vi "Buttons2.vi"() -> ()   [LabVIEW 2019]
panel:
  in  "LPB":bool
  in  "SPB":bool
  in  "LPA":bool
  in  "SPA":bool
  in  "Simulation":bool=TRUE
  in  "Array":bool[](array[boolean])=[FALSE, FALSE, FALSE, FALSE, FALSE, FALSE, FALSE, FALSE]
  in  "B":bool
  in  "A":bool
  in  "Exit":bool
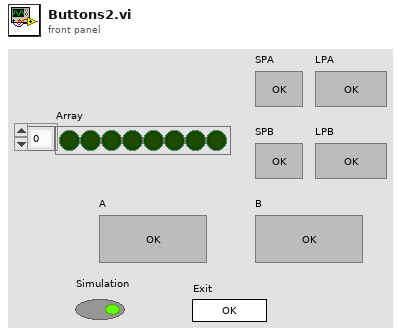
[diagram p1: front panel]
types:
  T1 = enum32{"Invalid", "Standard", "Closed", "Hidden", "Minimized", "Maximized"}
  T2 = enum32{"invalid app kind", "Development System", "Run Time System", "Student Edition", "Embedded LabVIEW", "Evaluation", "Custom"}
  T3 = cluster{"Core":cluster{"Current VI Reference":refnum<vi>, "Close Panel on Exit?":bool}, "A":bool, "B":bool, "Array":bool[], "NA":i32, "NB":i32}
  T4 = cluster{"Current VI Reference":refnum<vi>, "Close Panel on Exit?":bool}
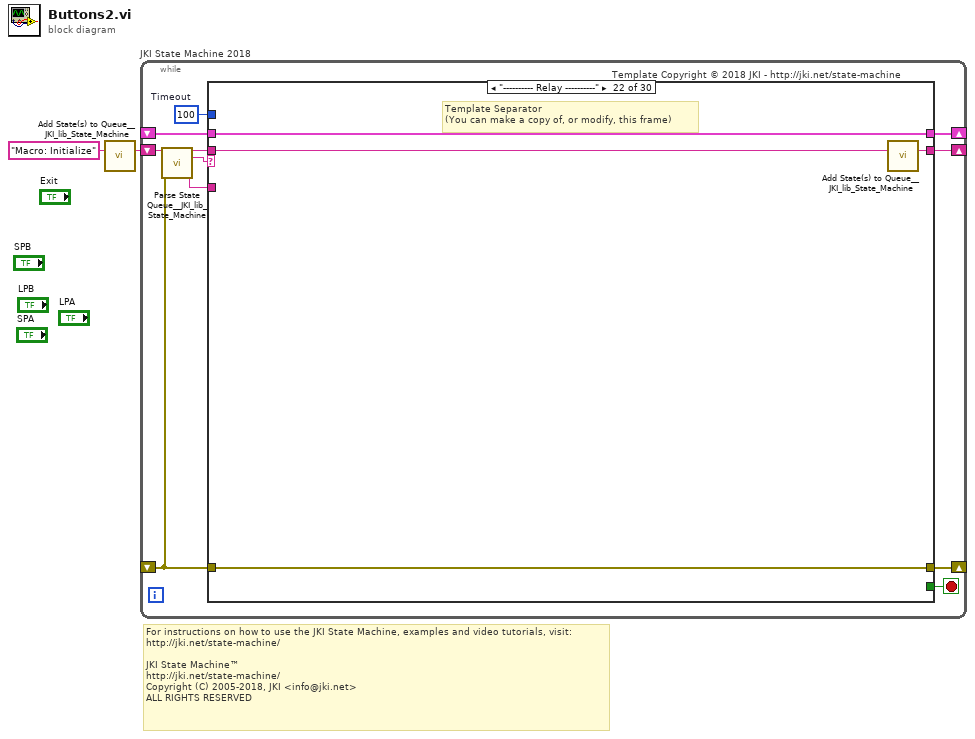
[diagram p0: block diagram]
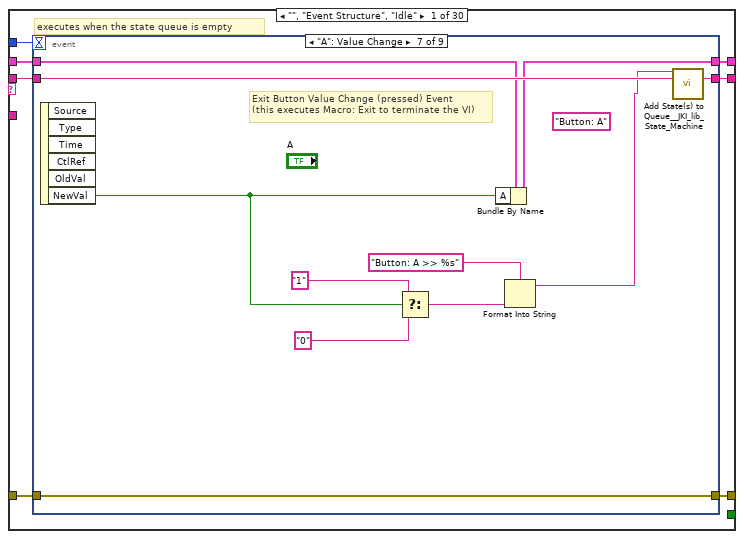
[diagram p2: hidden frame]
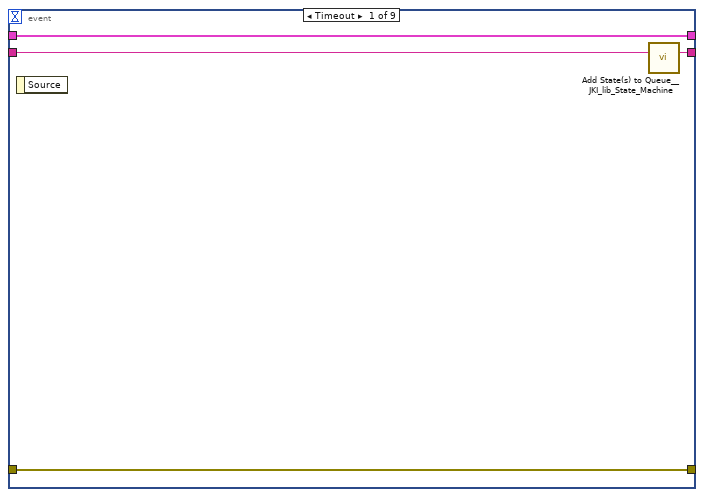
[diagram p3: hidden frame]
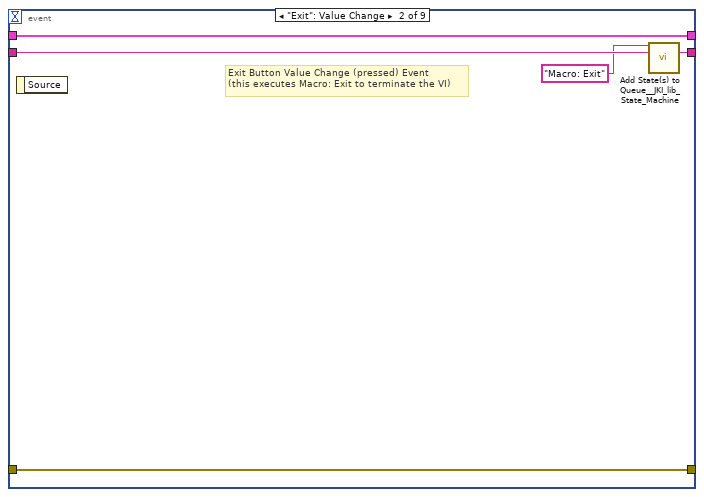
[diagram p4: hidden frame]
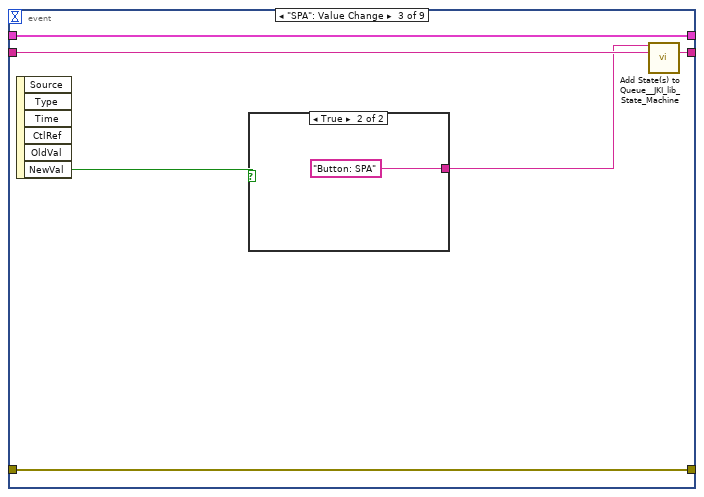
[diagram p5: hidden frame]
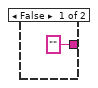
[diagram p6: hidden frame]
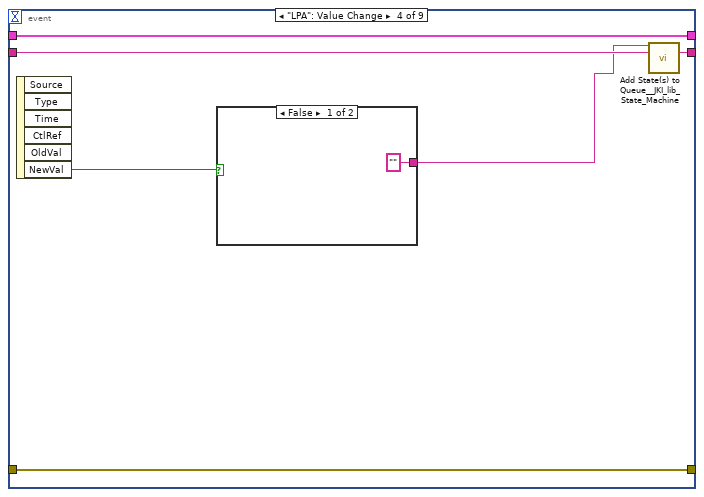
[diagram p7: hidden frame]
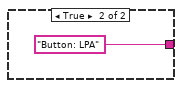
[diagram p8: hidden frame]
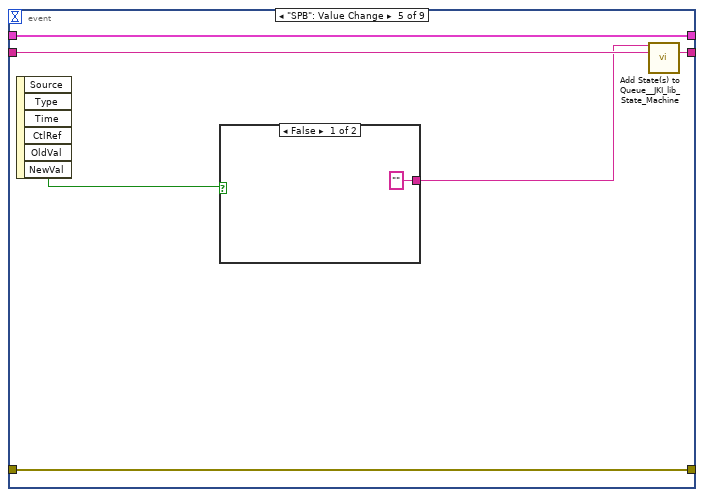
[diagram p9: hidden frame]
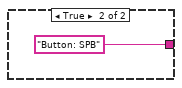
[diagram p10: hidden frame]
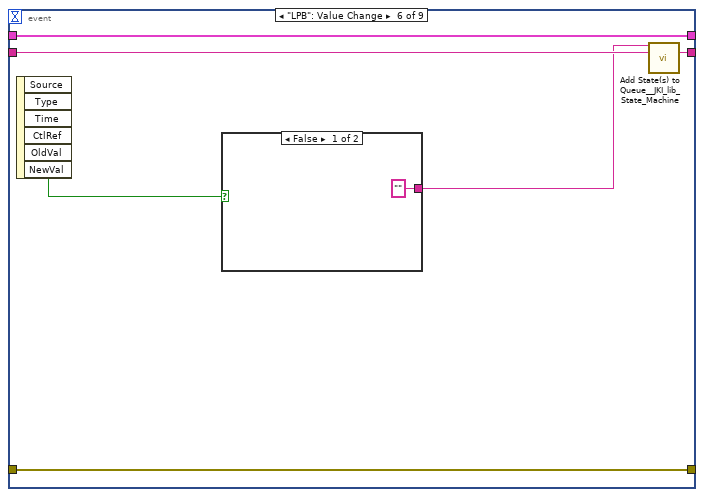
[diagram p11: hidden frame]
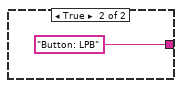
[diagram p12: hidden frame]
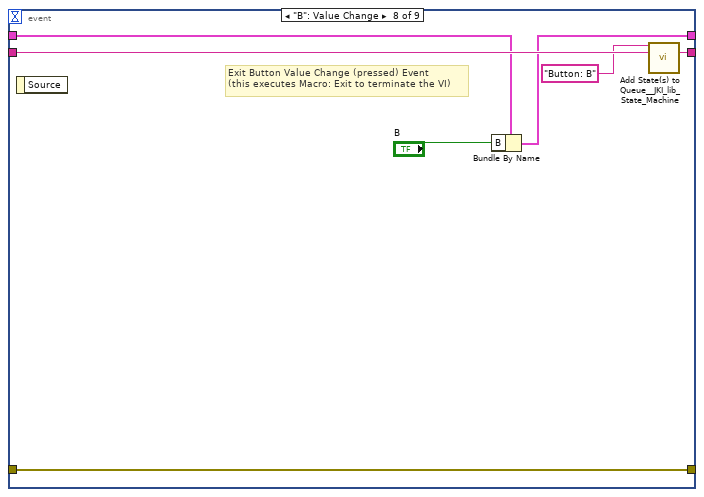
[diagram p13: hidden frame]
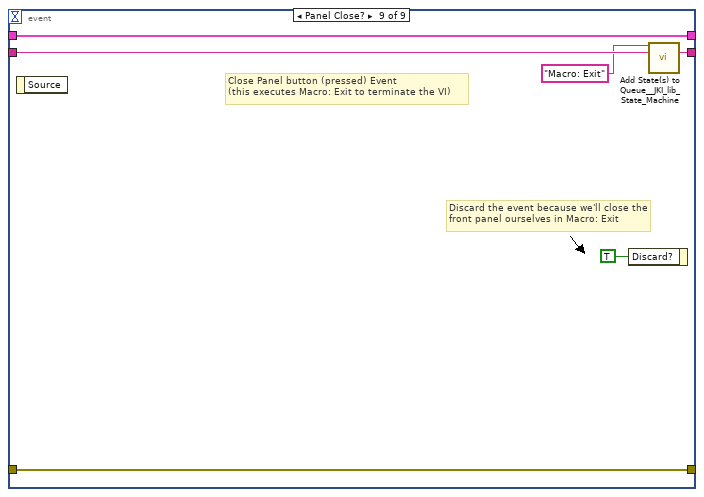
[diagram p14: hidden frame]
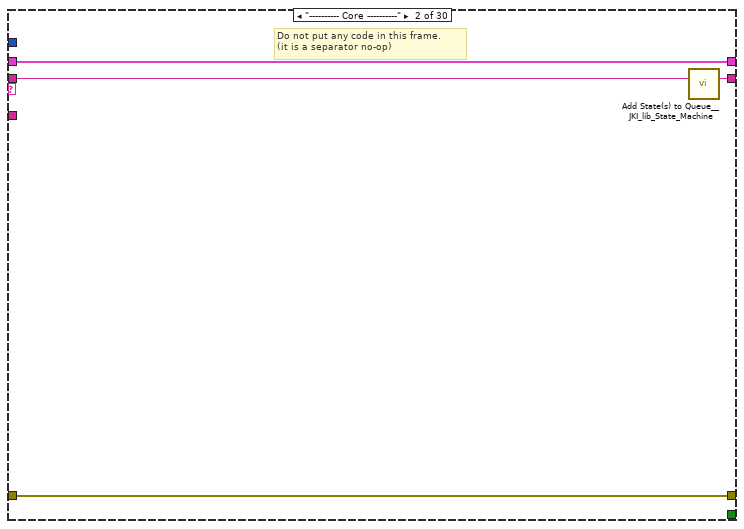
[diagram p15: hidden frame]
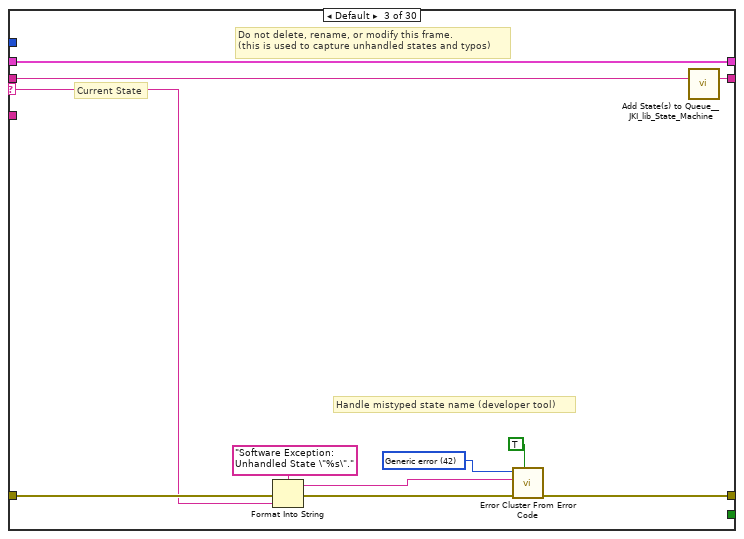
[diagram p16: hidden frame]
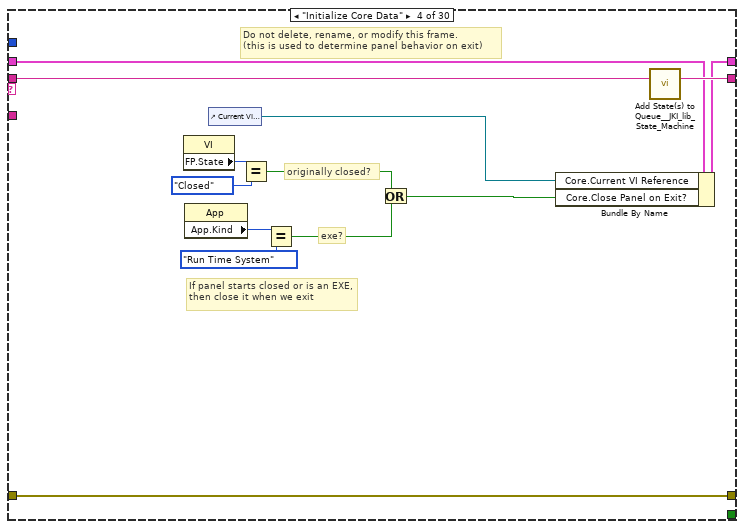
[diagram p17: hidden frame]
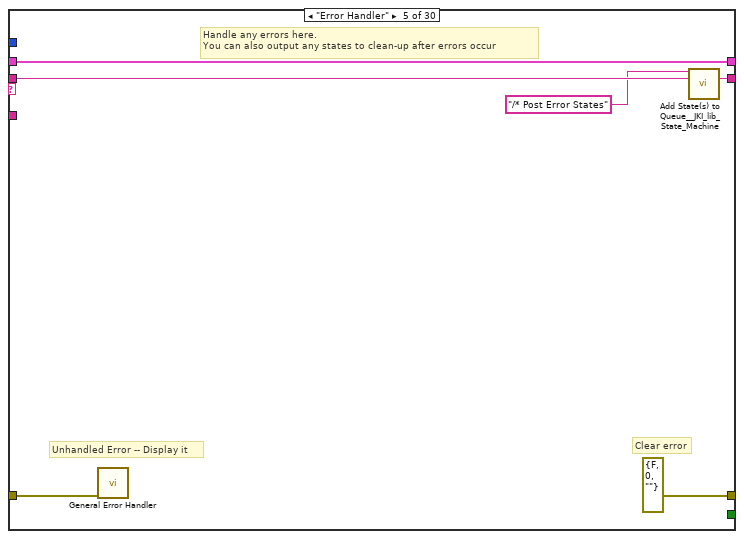
[diagram p18: hidden frame]
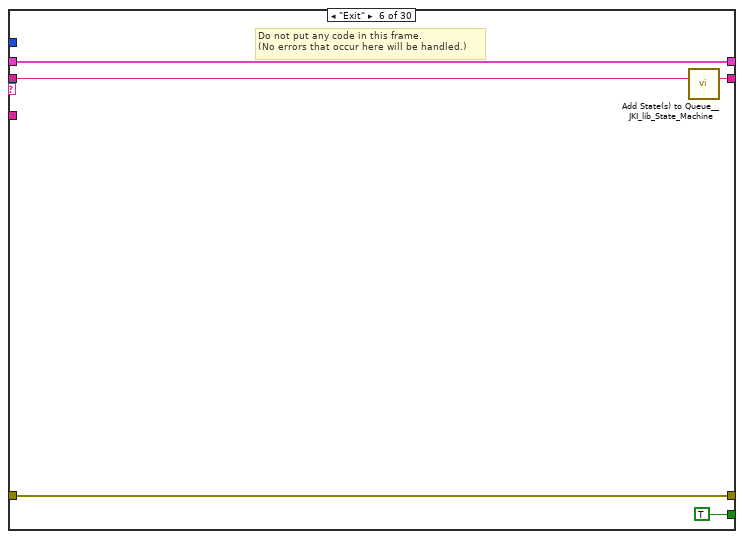
[diagram p19: hidden frame]
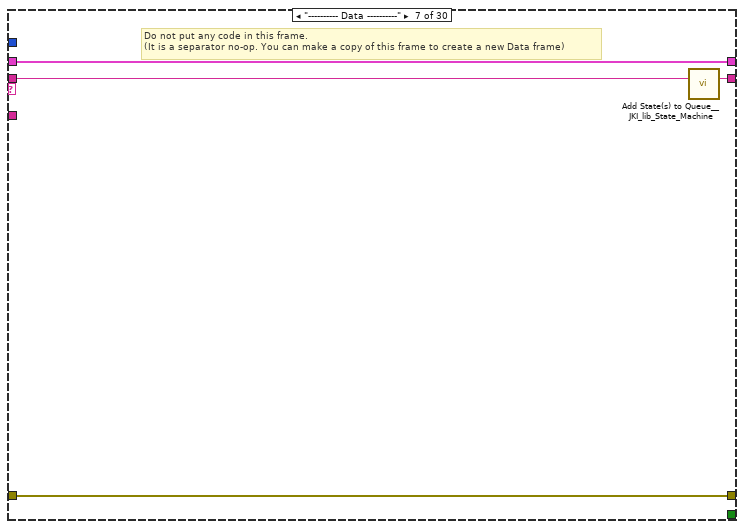
[diagram p20: hidden frame]
diagram:
  # "For instructions on how to use the JKI State Machine, examples and video tutorials, visit:\nhttp://jki.net/state-machine/\n\nJKI State Machine™\nhttp://jki.net/state-machine/\nCopyright (C) 2005-2018, JKI <info@jki.net>\nALL RIGHTS RESERVED"
  n1 = call <vilib>:"Add State(s) to Queue__JKI_lib_State_Machine.vi"("State(s) in (\"\")"="Macro: Initialize") -> ("States Out"=w2:string)  [unwired: 14 in]
  n2 = while "JKI State Machine 2018" {
    shift-right: [w7] -> _
    shift-left: _ -> [w6]
    shift-right: [w10] -> _
    shift-left: _ -> [w4]
    shift-right: [w9] -> _
    shift-left: w2 -> [w11]
    stop <- w8 stop-if-true
    w5 = 100  # Timeout
    # "Template Copyright © 2018 JKI - http://jki.net/state-machine"
    n3 = call <vilib>:"Parse State Queue__JKI_lib_State_Machine.vi"("State Queue"=w11, "Error In (no error)"=w4) -> ("Remaining States"=w12:string, "Current State"=w13:string, "Arguments"=w3:string)  [unwired: 11 in]
    n4 = case shown="\"---------- Relay ----------\"" w13 {
      selector: w13 -> [_ _ w90 _ _ _ _ _ _ _ _ _ _ _ _ _ _ _ _ _ _ _ _ _ _ _ _ _ _ _]
      tunnel: w12 -> [w20 w89 w94 w113 w119 w124 w128 w138 w144 w148 w152 w158 w169 w238 w243 w253 w257 w277 w299 w307 w314 w321 w327 w333 w339 w343 w348 w353 w358 w363]
      tunnel: w6 -> [w18 w86 w92 w106 w116 w122 w125 _ w139 w145 w150 w156 w165 w235 w240 w250 w254 w271 w293 w304 w311 w318 w325 w331 w337 w340 w345 w350 w355 w360]
      tunnel: [w17 w87 w96 w110 errorcluster {"status"=FALSE, "code"=0, "source"=""} ("error out") w121 w126 w135 w140 w146 w149 w154 w166 w236 w241 w251 w255 w275 w297 w305 w309 w319 w323 w329 w334 w341 w346 w351 w356 w361] -> w10
      tunnel: w4 -> [w16 w87 w95 w110 w115 w121 w126 w135 w141 w146 w149 w155 w167 w236 w241 w251 w255 w275 w297 w305 w308 w319 w324 w330 w335 w341 w346 w351 w356 w361]
      tunnel: [w19 w88 w93 w112 w118 w123 w127 w137 w143 w147 w151 w157 w168 w237 w242 w252 w256 w276 w298 w306 w313 w320 w326 w332 w338 w342 w347 w352 w357 w362] -> w9
      tunnel: [_ _ _ _ _ TRUE _ _ _ _ _ _ _ _ _ _ _ _ _ _ _ _ _ _ _ _ _ _ _ _] -> w8
      tunnel: [w15 w86 w92 w111 w116 w122 w125 w136 w139 w145 w150 w156 w165 w235 w240 w250 w254 w272 w294 w304 w311 w318 w325 w331 w337 w340 w345 w350 w355 w360] -> w7
      tunnel: w5 -> [w14 _ _ _ _ _ _ _ _ _ _ _ _ _ _ _ _ _ _ _ _ _ _ _ _ _ _ _ _ _]
      tunnel: w3 -> [_ _ _ _ _ _ _ _ _ _ _ w153 w163 _ _ _ _ w264 w286 w302 _ _ _ _ _ _ _ _ _ _]
      frame "", "Event Structure", "Idle" {
        # "executes when the state queue is empty"
        n5 = event shown="[6] \"A\": Value Change" {
          selector: _ -> [_ _ _ _ _ _ _ _ _]
          dyn-events: _ -> [_ _ _ _ _ _ _ _ _]
          timeout: w14 -> [_ _ _ _ _ _ _ _ _]
          tunnel: w20 -> [w24 w29 w35 w43 w51 w59 w72 w79 w85]
          tunnel: [w23 w28 w34 w42 w50 w58 w71 w78 w84] -> w19
          tunnel: w18 -> [w21 w26 w32 w40 w48 w56 w69 w73 w82]
          tunnel: [w22 w27 w33 w41 w49 w57 w70 w77 w83] -> w17
          tunnel: w16 -> [w22 w27 w33 w41 w49 w57 w70 w77 w83]
          tunnel: [w21 w26 w32 w40 w48 w56 w68 w74 w82] -> w15
          event Timeout {
            n6 = event-data() -> ()  [unwired: 1 in, 1 out]
            n7 = call <vilib>:"Add State(s) to Queue__JKI_lib_State_Machine.vi"("State(s) in (\"\")"=w24) -> ("States Out"=w23:string)  [unwired: 14 in]
          }
          event "Exit": Value Change {
            # "Exit Button Value Change (pressed) Event\n(this executes Macro: Exit to terminate the VI)"
            n8 = event-data() -> ()  [unwired: 1 in, 1 out]
            n9 = call <vilib>:"Add State(s) to Queue__JKI_lib_State_Machine.vi"("State(s) in Front (\"\")"="Macro: Exit", "State(s) in (\"\")"=w29) -> ("States Out"=w28:string)  [unwired: 13 in]
          }
          event "SPA": Value Change {
            n10 = event-data() -> ("NewVal"=w30:bool)  [unwired: 1 in, 5 out]
            n11 = case shown="True" w30 {
              tunnel: ["" "Button: SPA"] -> w31
              frame False {
              }
              frame True {
              }
            }
            n12 = call <vilib>:"Add State(s) to Queue__JKI_lib_State_Machine.vi"("State(s) in Front (\"\")"=w31, "State(s) in (\"\")"=w35) -> ("States Out"=w34:string)  [unwired: 13 in]
          }
          event "LPA": Value Change {
            n13 = event-data() -> ("NewVal"=w38:bool)  [unwired: 1 in, 5 out]
            n14 = case shown="False" w38 {
              tunnel: ["" "Button: LPA"] -> w39
              frame False {
              }
              frame True {
              }
            }
            n15 = call <vilib>:"Add State(s) to Queue__JKI_lib_State_Machine.vi"("State(s) in Front (\"\")"=w39, "State(s) in (\"\")"=w43) -> ("States Out"=w42:string)  [unwired: 13 in]
          }
          event "SPB": Value Change {
            n16 = event-data() -> ("NewVal"=w46:bool)  [unwired: 1 in, 5 out]
            n17 = case shown="False" w46 {
              tunnel: ["" "Button: SPB"] -> w47
              frame False {
              }
              frame True {
              }
            }
            n18 = call <vilib>:"Add State(s) to Queue__JKI_lib_State_Machine.vi"("State(s) in Front (\"\")"=w47, "State(s) in (\"\")"=w51) -> ("States Out"=w50:string)  [unwired: 13 in]
          }
          event "LPB": Value Change {
            n19 = event-data() -> ("NewVal"=w54:bool)  [unwired: 1 in, 5 out]
            n20 = case shown="False" w54 {
              tunnel: ["" "Button: LPB"] -> w55
              frame False {
              }
              frame True {
              }
            }
            n21 = call <vilib>:"Add State(s) to Queue__JKI_lib_State_Machine.vi"("State(s) in Front (\"\")"=w55, "State(s) in (\"\")"=w59) -> ("States Out"=w58:string)  [unwired: 13 in]
          }
          event "A": Value Change {
            (unwired) "Button: A"
            # "Exit Button Value Change (pressed) Event\n(this executes Macro: Exit to terminate the VI)"
            n22 = event-data() -> ("NewVal"=w67:bool)  [unwired: 1 in, 5 out]
            n23 = Select(t="1", s=w67, f="0") -> (s? t:f=w65:string)
            n24 = Bundle By Name(cluster=w69, "A"=w67) -> (w68:T3)
            n25 = Format Into String(format string="Button: A >> %s", w65) -> (resulting string=w62:string)  [unwired: 2 in, 1 out]
            n26 = call <vilib>:"Add State(s) to Queue__JKI_lib_State_Machine.vi"("State(s) in Front (\"\")"=w62, "State(s) in (\"\")"=w72) -> ("States Out"=w71:string)  [unwired: 13 in]
          }
          event "B": Value Change {
            # "Exit Button Value Change (pressed) Event\n(this executes Macro: Exit to terminate the VI)"
            n27 = event-data() -> ()  [unwired: 1 in, 1 out]
            n28 = Bundle By Name(cluster=w73, "B"="B") -> (w74:T3)
            n29 = call <vilib>:"Add State(s) to Queue__JKI_lib_State_Machine.vi"("State(s) in Front (\"\")"="Button: B", "State(s) in (\"\")"=w79) -> ("States Out"=w78:string)  [unwired: 13 in]
          }
          event Panel Close? {
            # "Discard the event because we'll close the front panel ourselves in Macro: Exit"
            # "Close Panel button (pressed) Event\n(this executes Macro: Exit to terminate the VI)"
            n30 = event-data() -> ()  [unwired: 1 in, 1 out]
            n31 = event-data("Discard?"=TRUE) -> ()  [unwired: 1 in, 1 out]
            n32 = call <vilib>:"Add State(s) to Queue__JKI_lib_State_Machine.vi"("State(s) in Front (\"\")"="Macro: Exit", "State(s) in (\"\")"=w85) -> ("States Out"=w84:string)  [unwired: 13 in]
          }
        }
      }
      frame "---------- Core ----------" {
        # "Do not put any code in this frame.\n(it is a separator no-op)"
        n33 = call <vilib>:"Add State(s) to Queue__JKI_lib_State_Machine.vi"("State(s) in (\"\")"=w89) -> ("States Out"=w88:string)  [unwired: 14 in]
      }
      frame Default {
        w99 = 42 items=["No error", "Argument error", "Memory is full", "Out of zone", "End of file", "File already open", "Generic file I/O error", "File not found", "File permission error", "Disk is full", "Duplicate path", "Too many files open", "System feature not enabled", "Resource file not found", "Cannot add resource", "Resource not found", "Image not found", "Image memory error", "Pen does not exist", "Config type invalid", "Config token not found", "Config parse error", "Config memory error", "Bad external code format", "Bad external code offset", "External code not present", "Null window", "Destroy window error", "Null menu", "Print aborted", "Bad print record", "Print driver error", "Windows error during printing", "Memory error during printing", "Print dialog error", "Generic print error", "Invalid device refnum", "Device not found", "Device parameter error", "Device unit error", "Cannot open device", "Device call aborted", "Generic error", "Cancelled by user", "Object ID too low", "Object ID too high", "Object not in heap", "Unknown heap", "Unknown object (invalid DefProc)", "Unknown object (DefProc not in table)", "Message out of range", "Invalid (null) method", "Unknown message", "Manager call not supported", "Bad address", "Network operation in progress", "Network operation timed out", "Connection is busy", "Network attribute not supported", "Network error", "Address in use", "System out of memory", "Connection aborted", "Connection refused", "Not connected", "Already connected", "Connection closed", "Initialization error (interapplication manager)", "Bad occurrence", "Wait on unbound occurrence handler", "Occurrence queue overflow", "Datalog type conflict", "Unused", "Unrecognized type (interapplication manager)", "Memory corrupt", "Failed to make temporary DLL", "Old CIN version", "Drag socket not found", "Failed to load drop-object", "Failed to register OLE object", "Failed to release OLE object", "Format specifier type mismatch", "Unknown format specifier", "Too few format specifiers", "Too many format specifiers", "Scan failed", "Newer CIN version", "Error converting to variant", "Runtime menu error", "Password tampered", "Variant attribute not found", "Incompatible variant data type", "Event data is not available", "Event Store is not present", "Occurrence is not found", "Event Queue is not created", "Event info is not available", "Refnum passed is NULL", "Error retrieving Class GUID", "Error retrieving CoClass GUID", "Error retrieving TypeLib GUID.", "Bad built application magic bytes.", "Specific driver is different from the specific driver associated with the Logical Name.", "There is no session opened to the class driver.", "Max Error", "MAX - Error with config objects", "MAX - Error loading configuration", "MAX - Group not supported"]
        # "Current State"
        # "Do not delete, rename, or modify this frame.\n(this is used to capture unhandled states and typos)"
        # "Handle mistyped state name (developer tool)"
        n34 = Format Into String(format string="Software Exception: Unhandled State \"%s\"." ("message"), error in=w95, w90) -> (resulting string=w98:string, error out=w97:errorcluster)  [unwired: 1 in]
        n35 = call <vilib>:"Error Cluster From Error Code.vi"("show call chain? (False)"=TRUE, "error in (no error)"=w97, "error message (\"\")"=w98, "error code (0)"=w99) -> ("error out"=w96:errorcluster)  [unwired: 5 in]
        n36 = call <vilib>:"Add State(s) to Queue__JKI_lib_State_Machine.vi"("State(s) in (\"\")"=w94) -> ("States Out"=w93:string)  [unwired: 14 in]
      }
      frame "Initialize Core Data" {
        # "Do not delete, rename, or modify this frame.\n(this is used to determine panel behavior on exit)"
        # "originally closed?"
        # "exe?"
        # "If panel starts closed or is an EXE, then close it when we exit"
        n37 = property class="VI"() -> ("FP.State"=w103:T1)  [unwired: 2 in, 2 out]
        n38 = property class="App"() -> ("App.Kind"=w109:T2)  [unwired: 2 in, 2 out]
        n39 = control-ref of="Current VI Reference"() -> (w104:refnum<vi>)
        n40 = Equal?(x=w103, y=T1."Closed" ("Front Panel Window:State")) -> (x = y?=w101:bool)
        n41 = Equal?(x=w109, y=T2."Run Time System" ("Application:Kind")) -> (x = y?=w107:bool)
        n42 = Or(x=w101, y=w107) -> (x .or. y?=w105:bool)
        n43 = Bundle By Name(cluster=w106, "Core.Current VI Reference"=w104, "Core.Close Panel on Exit?"=w105) -> (w111:T3)
        n44 = call <vilib>:"Add State(s) to Queue__JKI_lib_State_Machine.vi"("State(s) in (\"\")"=w113) -> ("States Out"=w112:string)  [unwired: 14 in]
      }
      frame "Error Handler" {
        # "Unhandled Error -- Display it"
        # "Handle any errors here.\nYou can also output any states to clean-up after errors occur"
        # "Clear error"
        n45 = call <vilib>:"General Error Handler.vi"("error in (no error)"=w115) -> ()  [unwired: 10 in, 5 out]
        n46 = call <vilib>:"Add State(s) to Queue__JKI_lib_State_Machine.vi"("State(s) in Front (\"\")"="/* Post Error States", "State(s) in (\"\")"=w119) -> ("States Out"=w118:string)  [unwired: 13 in]
      }
      frame "Exit" {
        # "Do not put any code in this frame.\n(No errors that occur here will be handled.)"
        n47 = call <vilib>:"Add State(s) to Queue__JKI_lib_State_Machine.vi"("State(s) in (\"\")"=w124) -> ("States Out"=w123:string)  [unwired: 14 in]
      }
      frame "---------- Data ----------" {
        # "Do not put any code in this frame.\n(It is a separator no-op. You can make a copy of this frame to create a new Data frame)"
        n48 = call <vilib>:"Add State(s) to Queue__JKI_lib_State_Machine.vi"("State(s) in (\"\")"=w128) -> ("States Out"=w127:string)  [unwired: 14 in]
      }
      frame "Data: Initialize" {
        w129 = 4  # NB
        w130 = 2  # NA
        w132 = TRUE  # B
        w133 = T4 {"Current VI Reference"=refnum, "Close Panel on Exit?"=FALSE}  # Core
        w134 = TRUE  # A
        # "do not delete - used by framework"
        # "Initialize the shift-register data, here.\n(data names are defined by what you wire into the bundle function)"
        n49 = Bundle("Core"=w133, "A"=w134, "B"=w132, "Array"="Array", "NA"=w130, "NB"=w129) -> (w136:T3)  [unwired: 1 in]
        n50 = call <vilib>:"Add State(s) to Queue__JKI_lib_State_Machine.vi"("State(s) in (\"\")"=w138) -> ("States Out"=w137:string)  [unwired: 14 in]
      }
      frame "Data: Cleanup" {
        # "Cleanup any data and references, here.\n(this is called automatically, by the Macro: Exit)"
        n51 = Unbundle By Name(w139) -> ("Core.Current VI Reference"=w142:refnum<vi>)
        n52 = Close Reference(reference=w142, error in (no error)=w141) -> (error out=w140:errorcluster)
        n53 = call <vilib>:"Add State(s) to Queue__JKI_lib_State_Machine.vi"("State(s) in (\"\")"=w144) -> ("States Out"=w143:string)  [unwired: 14 in]
      }
      frame "---------- UI ----------" {
        # "Do not put any code in this frame.\n(It is a separator no-op. You can make a copy of this frame to create a new UI frame)"
        n54 = call <vilib>:"Add State(s) to Queue__JKI_lib_State_Machine.vi"("State(s) in (\"\")"=w148) -> ("States Out"=w147:string)  [unwired: 14 in]
      }
      frame "UI: Initialize" {
        # "Initialize the User Interface, here.\n(this is called automatically, by the Macro: Init)"
        n55 = call <vilib>:"Add State(s) to Queue__JKI_lib_State_Machine.vi"("State(s) in (\"\")"=w152) -> ("States Out"=w151:string)  [unwired: 14 in]
      }
      frame "UI: Cursor Set" {
        # "Set and Unset Cursor Busy.\n(Usage: \"UI: Cursor Set >> Busy|Idle\")"
        n56 = case shown="\"Busy\"" w153 {
          tunnel: w155 -> [w160 w162]
          tunnel: [w159 w161] -> w154
          frame "Idle", Default {
            n57 = call <vilib>:"Unset Busy.vi"("error in (no error)"=w160) -> ("error out"=w159:errorcluster)  [unwired: 10 in]
          }
          frame "Busy" {
            n58 = call <vilib>:"Set Busy.vi"("error in (no error)"=w162) -> ("error out"=w161:errorcluster)  [unwired: 9 in, 1 out]
          }
        }
        n59 = call <vilib>:"Add State(s) to Queue__JKI_lib_State_Machine.vi"("State(s) in (\"\")"=w158) -> ("States Out"=w157:string)  [unwired: 14 in]
      }
      frame "UI: Front Panel State" {
        # "Argument"
        # "Set Front Panel Open or Closed\n(Usage: \"UI: Front Panel State >> Open|Close\")"
        n60 = Unbundle By Name(w165) -> ("Core.Current VI Reference"=w164:refnum<vi>)
        n61 = case shown="\"Minimize\", \"Minimized\"" w163 {
          tunnel: w167 -> [w175 w190 w201 w214 w227]
          tunnel: [w177 w191 w203 w216 w229] -> w166
          tunnel: w164 -> [w176 w188 w202 w215 w228]
          frame "Open", "Standard", Default {
            w170 = T1."Standard" ("State")
            n62 = property class="VI"(reference=w176, error in=w175) -> (reference out=w173:refnum<vi>, error out=w174:errorcluster, "FP.State"=w172:T1)
            n63 = Not Equal?(x=w172, y=w170) -> (x != y?=w171:bool)
            n64 = case shown="True" w171 {
              tunnel: [w181 w183] -> w177
              tunnel: w174 -> [w180 w183]
              tunnel: w173 -> [w179 _]
              tunnel: w170 -> [w178 _]
              frame True {
                n65 = invoke class="VI" method="FP.Open"(reference=w179, error in=w180, "Activate"=TRUE, "State"=w178) -> (error out=w181:errorcluster)  [unwired: 1 in, 4 out]
              }
              frame False {
              }
            }
          }
          frame "Close", "Closed" {
            n66 = property class="VI"(reference=w188, error in=w190) -> (reference out=w187:refnum<vi>, error out=w189:errorcluster, "FP.State"=w185:T1)
            n67 = Not Equal?(x=w185, y=T1."Closed" ("Front Panel Window:State")) -> (x != y?=w184:bool)
            n68 = case shown="True" w184 {
              tunnel: [w192 w195] -> w191
              tunnel: w189 -> [w192 w194]
              tunnel: w187 -> [_ w193]
              frame False {
              }
              frame True {
                n69 = invoke class="VI" method="FP.Close"(reference=w193, error in=w194) -> (error out=w195:errorcluster)  [unwired: 1 in, 2 out]
              }
            }
          }
          frame "Hidden", "Hide" {
            w196 = T1."Hidden" ("State")
            n70 = property class="VI"(reference=w202, error in=w201) -> (reference out=w199:refnum<vi>, error out=w200:errorcluster, "FP.State"=w198:T1)
            n71 = Not Equal?(x=w198, y=w196) -> (x != y?=w197:bool)
            n72 = case shown="True" w197 {
              tunnel: [w207 w208] -> w203
              tunnel: w200 -> [w206 w208]
              tunnel: w199 -> [w205 _]
              tunnel: w196 -> [w204 _]
              frame True {
                n73 = invoke class="VI" method="FP.Open"(reference=w205, error in=w206, "State"=w204) -> (error out=w207:errorcluster)  [unwired: 2 in, 4 out]
              }
              frame False {
              }
            }
          }
          frame "Minimize", "Minimized" {
            w209 = T1."Minimized" ("State")
            n74 = property class="VI"(reference=w215, error in=w214) -> (reference out=w212:refnum<vi>, error out=w213:errorcluster, "FP.State"=w211:T1)
            n75 = Not Equal?(x=w211, y=w209) -> (x != y?=w210:bool)
            n76 = case shown="True" w210 {
              tunnel: [w220 w221] -> w216
              tunnel: w213 -> [w219 w221]
              tunnel: w212 -> [w218 _]
              tunnel: w209 -> [w217 _]
              frame True {
                n77 = invoke class="VI" method="FP.Open"(reference=w218, error in=w219, "State"=w217) -> (error out=w220:errorcluster)  [unwired: 2 in, 4 out]
              }
              frame False {
              }
            }
          }
          frame "Maximize", "Maximized" {
            w222 = T1."Maximized" ("State")
            n78 = property class="VI"(reference=w228, error in=w227) -> (reference out=w225:refnum<vi>, error out=w226:errorcluster, "FP.State"=w224:T1)
            n79 = Not Equal?(x=w224, y=w222) -> (x != y?=w223:bool)
            n80 = case shown="True" w223 {
              tunnel: [w233 w234] -> w229
              tunnel: w226 -> [w232 w234]
              tunnel: w225 -> [w231 _]
              tunnel: w222 -> [w230 _]
              frame True {
                n81 = invoke class="VI" method="FP.Open"(reference=w231, error in=w232, "State"=w230) -> (error out=w233:errorcluster)  [unwired: 2 in, 4 out]
              }
              frame False {
              }
            }
          }
        }
        n82 = call <vilib>:"Add State(s) to Queue__JKI_lib_State_Machine.vi"("State(s) in (\"\")"=w169) -> ("States Out"=w168:string)  [unwired: 14 in]
      }
      frame "---------- Macro ----------" {
        # "Do not put any code in this frame.\n(It is a separator no-op. You can make a copy of this frame to create a new Macro frame)"
        n83 = call <vilib>:"Add State(s) to Queue__JKI_lib_State_Machine.vi"("State(s) in (\"\")"=w238) -> ("States Out"=w237:string)  [unwired: 14 in]
      }
      frame "Macro: Initialize" {
        # "Initialization Macro\n(This is called once, when the VI starts)"
        n84 = call <vilib>:"Add State(s) to Queue__JKI_lib_State_Machine.vi"("State(s) in Front (\"\")"="Data: Initialize\nInitialize Core Data\nUI: Initialize\nUI: Front Panel State >> Open", "State(s) in (\"\")"=w243) -> ("States Out"=w242:string)  [unwired: 13 in]
      }
      frame "Macro: Exit" {
        # "Exit Macro\n(This is called once, when the VI exits)"
        n85 = Unbundle By Name(w250) -> ("Core.Close Panel on Exit?"=w249:bool)
        n86 = Select(t="UI: Front Panel State >> Close", s=w249, f="") -> (s? t:f=w246:string)
        n87 = call <vilib>:"Add State(s) to Queue__JKI_lib_State_Machine.vi"("State(s) in (\"\")"=w246, "State(s) at Back (\"\")"="Data: Cleanup\nExit") -> ("States Out"=w244:string)  [unwired: 13 in]
        n88 = call <vilib>:"Add State(s) to Queue__JKI_lib_State_Machine.vi"("State(s) in Front (\"\")"=w244, "State(s) in (\"\")"=w253) -> ("States Out"=w252:string)  [unwired: 13 in]
      }
      frame "---------- Press ----------" {
        # "Template Separator\n(You can make a copy of, or modify, this frame)"
        n89 = call <vilib>:"Add State(s) to Queue__JKI_lib_State_Machine.vi"("State(s) in (\"\")"=w257) -> ("States Out"=w256:string)  [unwired: 14 in]
      }
      frame "Button: A" {
        # "Your code here.\n(You can make a copy of, or modify, this frame)"
        n90 = Decimal String To Number(string=w264) -> (number=w267:i32)  [unwired: 2 in, 1 out]
        n91 = Empty String/Path?(string/path=w264) -> (empty?=w268:bool)
        n92 = Equal To 0?(x=w267) -> (x = 0?=w266:bool)
        n93 = Not(x=w266) -> (.not. x?=w265:bool)
        n94 = Unbundle By Name(w271) -> ("NA"=w273:i32, "A"=w269:bool, "Array"=w274:bool[])
        n95 = case shown="True" w268 {
          tunnel: [w278 w279] -> w261
          tunnel: w269 -> [_ w279]
          tunnel: w265 -> [w278 _]
          frame False {
          }
          frame True {
          }
        }
        n96 = Replace Array Subset(array=w274, new element=w261, index=w273) -> (w270:bool[])
        n97 = Bundle By Name(cluster=w271, "Array"=w270) -> (w272:T3)
        n98 = Select(t="Relay: discharge tip", s=w261, f="Relay: open resistance") -> (s? t:f=w260:string)
        n99 = call <vilib>:"Add State(s) to Queue__JKI_lib_State_Machine.vi"("State(s) in Front (\"\")"="Button: Display", "State(s) at Back (\"\")"=w260) -> ("States Out"=w258:string)  [unwired: 13 in]
        n100 = call <vilib>:"Add State(s) to Queue__JKI_lib_State_Machine.vi"("State(s) in Front (\"\")"=w258, "State(s) in (\"\")"=w277) -> ("States Out"=w276:string)  [unwired: 13 in]
      }
      frame "Button: B" {
        # "Your code here.\n(You can make a copy of, or modify, this frame)"
        n101 = Decimal String To Number(string=w286) -> (number=w289:i32)  [unwired: 2 in, 1 out]
        n102 = Empty String/Path?(string/path=w286) -> (empty?=w290:bool)
        n103 = Equal To 0?(x=w289) -> (x = 0?=w288:bool)
        n104 = Not(x=w288) -> (.not. x?=w287:bool)
        n105 = Unbundle By Name(w293) -> ("NB"=w295:i32, "B"=w291:bool, "Array"=w296:bool[])
        n106 = case shown="True" w290 {
          tunnel: [w300 w301] -> w280
          tunnel: w291 -> [_ w301]
          tunnel: w287 -> [w300 _]
          frame False {
          }
          frame True {
          }
        }
        n107 = Replace Array Subset(array=w296, new element=w280, index=w295) -> (w292:bool[])
        n108 = Bundle By Name(cluster=w293, "Array"=w292) -> (w294:T3)
        n109 = Select(t="Relay: 0 ohms", s=w280, f="Relay: open resistance") -> (s? t:f=w283:string)
        n110 = call <vilib>:"Add State(s) to Queue__JKI_lib_State_Machine.vi"("State(s) in Front (\"\")"="Button: Display", "State(s) at Back (\"\")"=w283) -> ("States Out"=w281:string)  [unwired: 13 in]
        n111 = call <vilib>:"Add State(s) to Queue__JKI_lib_State_Machine.vi"("State(s) in Front (\"\")"=w281, "State(s) in (\"\")"=w299) -> ("States Out"=w298:string)  [unwired: 13 in]
      }
      frame "Button: Wait" {
        # "Template Separator\n(You can make a copy of, or modify, this frame)"
        n112 = Decimal String To Number(string=w302) -> (number=w303:i32)  [unwired: 2 in, 1 out]
        n113 = Wait (ms)(milliseconds to wait=w303) -> ()  [unwired: 1 out]
        n114 = call <vilib>:"Add State(s) to Queue__JKI_lib_State_Machine.vi"("State(s) in (\"\")"=w307) -> ("States Out"=w306:string)  [unwired: 14 in]
      }
      frame "Button: Display" {
        # "Your code here.\n(You can make a copy of, or modify, this frame)"
        n115 = Unbundle By Name(w311) -> ("Array"=w312:bool[])
        n116 = case shown="True" "Simulation" {
          tunnel: w312 -> [_ w317]
          tunnel: [w315 w316] -> w309
          tunnel: w308 -> [w315 w316]
          frame False {
          }
          frame True {
            n117 = local write "Array"(w317) -> ()
          }
        }
        n118 = call <vilib>:"Add State(s) to Queue__JKI_lib_State_Machine.vi"("State(s) in (\"\")"=w314) -> ("States Out"=w313:string)  [unwired: 14 in]
      }
      frame "---------- Relay ----------" {
        # "Template Separator\n(You can make a copy of, or modify, this frame)"
        n119 = call <vilib>:"Add State(s) to Queue__JKI_lib_State_Machine.vi"("State(s) in (\"\")"=w321) -> ("States Out"=w320:string)  [unwired: 14 in]
      }
      frame "Relay: discharge tip" {
        # "discharge = 2\n0 ohms = 8\nopen = 0"
        # "Template Separator\n(You can make a copy of, or modify, this frame)"
        n120 = call "Heater_D2XX.vi"("error in (no error)"=w324, "Numeric"=2) -> ("error out"=w323:errorcluster)  [unwired: 9 in]
        n121 = call <vilib>:"Add State(s) to Queue__JKI_lib_State_Machine.vi"("State(s) in (\"\")"=w327) -> ("States Out"=w326:string)  [unwired: 14 in]
      }
      frame "Relay: 0 ohms" {
        # "discharge = 2\n0 ohms = 8\nopen = 0"
        # "Template Separator\n(You can make a copy of, or modify, this frame)"
        n122 = call "Heater_D2XX.vi"("error in (no error)"=w330, "Numeric"=8) -> ("error out"=w329:errorcluster)  [unwired: 9 in]
        n123 = call <vilib>:"Add State(s) to Queue__JKI_lib_State_Machine.vi"("State(s) in (\"\")"=w333) -> ("States Out"=w332:string)  [unwired: 14 in]
      }
      frame "Relay: open resistance" {
        # "discharge = 2\n0 ohms = 8\nopen = 0"
        # "Template Separator\n(You can make a copy of, or modify, this frame)"
        n124 = call "Heater_D2XX.vi"("error in (no error)"=w335, "Numeric"=0) -> ("error out"=w334:errorcluster)  [unwired: 9 in]
        n125 = call <vilib>:"Add State(s) to Queue__JKI_lib_State_Machine.vi"("State(s) in (\"\")"=w339) -> ("States Out"=w338:string)  [unwired: 14 in]
      }
      frame "---------- Button ----------" {
        # "Template Separator\n(You can make a copy of, or modify, this frame)"
        n126 = call <vilib>:"Add State(s) to Queue__JKI_lib_State_Machine.vi"("State(s) in (\"\")"=w343) -> ("States Out"=w342:string)  [unwired: 14 in]
      }
      frame "Button: SPA" {
        # "Template Separator\n(You can make a copy of, or modify, this frame)"
        n127 = call <vilib>:"Add State(s) to Queue__JKI_lib_State_Machine.vi"("State(s) in Front (\"\")"="Button: A >> 1\nRelay: discharge tip\nButton: Wait >> 1\nRelay: open resistance\nButton: A >> 0" ("State(s) in Front (\"\")"), "State(s) in (\"\")"=w348) -> ("States Out"=w347:string)  [unwired: 13 in]
      }
      frame "Button: LPA" {
        # "Template Separator\n(You can make a copy of, or modify, this frame)"
        n128 = call <vilib>:"Add State(s) to Queue__JKI_lib_State_Machine.vi"("State(s) in Front (\"\")"="Button: A >> 1\nRelay: discharge tip\nButton: Wait >> 5000\nRelay: open resistance\nButton: A >> 0" ("State(s) in Front (\"\")"), "State(s) in (\"\")"=w353) -> ("States Out"=w352:string)  [unwired: 13 in]
      }
      frame "Button: SPB" {
        # "Template Separator\n(You can make a copy of, or modify, this frame)"
        n129 = call <vilib>:"Add State(s) to Queue__JKI_lib_State_Machine.vi"("State(s) in Front (\"\")"="Button: B >> 1\nRelay: 0 ohms\nButton: Wait >> 1\nRelay: open resistance\nButton: B >> 0" ("State(s) in Front (\"\")"), "State(s) in (\"\")"=w358) -> ("States Out"=w357:string)  [unwired: 13 in]
      }
      frame "Button: LPB" {
        # "Template Separator\n(You can make a copy of, or modify, this frame)"
        n130 = call <vilib>:"Add State(s) to Queue__JKI_lib_State_Machine.vi"("State(s) in Front (\"\")"="Button: B >> 1\nRelay: 0 ohms\nButton: Wait >> 5000\nRelay: open resistance\nButton: B >> 0" ("State(s) in Front (\"\")"), "State(s) in (\"\")"=w363) -> ("States Out"=w362:string)  [unwired: 13 in]
      }
    }
  }
